vi "ControllerUsage.vi"() -> ()   [LabVIEW 2017]
uses:
  <vilib>/rvi/Emulation/niFpgaGetClockAttributes.vi
  <vilib>/rvi/Emulation/niFpgaSctlEmulationGetInTimedLoop.vi
  <vilib>/rvi/Emulation/niFpgaEmulationReportErrorSimple.vi
  <vilib>/rvi/Emulation/niFpgaCriticalErrorInLSC.vi
  FPGA/BuckBoost.lvlib
panel:
  out "output":sgl[](array[numeric])
  in  "I_procVar":sgl[](array[numeric])=[0.0, 0.0, 0.0, 0.0]
  in  "I_setpt":sgl format="%#_13g"
  # "Device Utilization\n---------------------------\nTotal Slices: 35.0% (4654 out of 13300)\nSlice Registers: 11.7% (12443 out of 106400)\nSlice LUTs: 24.8% (13200 out of 53200)\nBlock RAMs: 3.6% (5 out of 140)\nDSP48s: 1.8% (4 out of 220)"
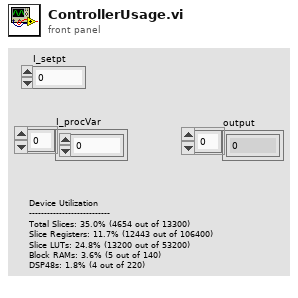
[diagram p1: front panel]
types:
  T1 = typedef "BuckBoost.lvlib/contSettings.ctl" = cluster{"numberOfInterleaves":refnum<k21>, "rampRate":refnum<k21>, "manualInput":refnum<k21>, "perturbAmp":refnum<k21>, "perturbAngleInc":refnum<k21>, "reset":refnum<k21>, "state":refnum<k21>, "gains":refnum<k21>, "Currents":refnum<k21>}
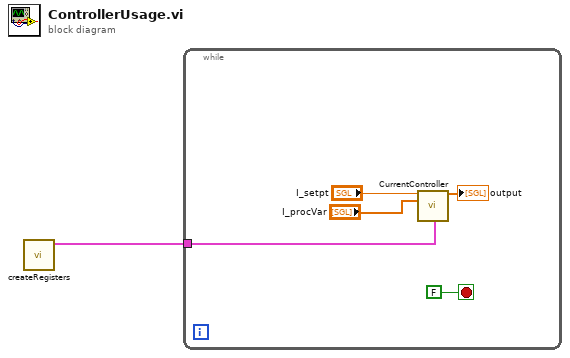
[diagram p0: block diagram]
diagram:
  n1 = call "createRegisters.vi"() -> ("settingsReg"=w1:T1)  [unwired: 10 in, 1 out]
  n2 = while {
    tunnel: w1 -> [w2]
    stop <- FALSE stop-if-true
    n3 = call "CurrentController.vi"("I_setpt"="I_setpt", "I_procVar"="I_procVar", "settings"=w2) -> ("output"=→"output":sgl[])  [unwired: 11 in, 1 out]
  }
